vi "PH_PPPA_PowerUnit.ProcEvents.vi"(0 "i ref in":refnum<vi>, 5 "error in (no error)":errorcluster) -> (14 "i ref out":refnum<vi>, 19 "error out":errorcluster)   [LabVIEW 2014, in "PH_PPPA_PowerUnit.lvlib"]
doc: "This method is used to define the events the object will listen to. Add your own events here."
uses:
  PH_PPPA_PowerUnit.lvlib
  CS_Core/BaseProcess/BaseProcess.event definition.ctl
  CS_Core/CAEObj/CAEObj.event definition.ctl
  CS_Core/BaseProcess/BaseProcess.descriptor string definition.ctl
  PH_Basics/PH_PP_Common/PH_PP_Common.Trigger Tags.ctl
  PH_Devices/PH_Beckhoff_PP_PU/PH_Beckhoff_PP_PU.RR Tags.ctl
  PH_Basics/PH_Common/DIM/PH_DIM.Event Declarer.ctl
  PH_Devices/PH_Beckhoff_PP_Control/PH_Beckhoff_PP_Control.PP Mercury Tags.ctl
  PH_Basics/PH_PP_Common/PH_PP_Common.PSU Tags.ctl
  PH_Basics/PH_PP_Common/PH_PP_Common.PUs.ctl
  PH_Devices/PH_Beckhoff_PP_PU/PH_Beckhoff_PP_PU.Igni Tags.ctl
  CS_Core/BaseProcess/BaseProcess.lvlib
  CS_Core/CAEObj/CAEObj.lvlib
  PH_Basics/PH_Common/PH_Common.lvlib
  PH_Basics/PH_PP_Common/PH_PP_Common.lvlib
  PH_Devices/PH_Beckhoff_PP_PU/PH_Beckhoff_PP_PU.lvlib
  PH_Devices/PH_Beckhoff_PP_Control/PH_Beckhoff_PP_Control.lvlib
  PH_Basics/PH_PowerUnit_BaseClass/PH_PowerUnit_BaseClass.lvlib
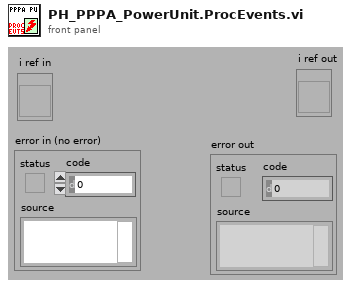
[diagram p1: front panel]
types:
  T1 = typedef "PH_Beckhoff_PP_PU.lvlib/PH_Beckhoff_PP_PU.RR Tags.ctl" = enum16{"open", "closed", "close", "Status"}
  T2 = typedef "BaseProcess.lvlib/BaseProcess.event definition.ctl" = cluster{"CAEEvtDef":T3, "Data Descriptor":T4}
  T3 = typedef "CAEObj.lvlib/CAEObj.event definition.ctl" = cluster{"URL":string, "enable":bool, "ignoreResID":bool}
  T4 = typedef "BaseProcess.lvlib/BaseProcess.descriptor string definition.ctl" = string
  T5 = typedef "PH_Common.lvlib/PH_DIM.Event Declarer.ctl" = cluster{"Service Name":string, "Selector":string}
  T6 = typedef "PH_Beckhoff_PP_Control.lvlib/PH_Beckhoff_PP_Control.PP Mercury Tags.ctl" = enum16{"Device-on", "Alarm", "on-since", "Concentration", "Status"}
  T7 = typedef "PH_PP_Common.lvlib/PH_PP_Common.PSU Tags.ctl" = enum16{"voltage-indicator", "peak-detect", "current", "voltage", "inihibit-indicator", "end-of-charge", "HV-on-indicator", "overtemperature", "interlock-indicator", "load-fault", "sum-fault", "HV-off-indicator", "DC-ok", "inhibit", "HV-on", "interlock", "reset", "Status", "Limits"}
  T8 = typedef "PH_PP_Common.lvlib/PH_PP_Common.PUs.ctl" = enum16{"no Info", "PA-19mm-1", "PA-19mm-2", "PA-45mm-PILC", "PA-45mm-MAIN", "MA-PU-1", "MA-PU-2", "MA-PU-3", "MA-PU-4", "MA-PU-5", "MA-PU-6", "MA-FR", "MA-PILC", "PA-45mm-DP"}
  T9 = typedef "PH_Beckhoff_PP_PU.lvlib/PH_Beckhoff_PP_PU.Igni Tags.ctl" = enum16{"heating-on", "water-on", "Device-on", "Status"}
  T10 = typedef "PH_PP_Common.lvlib/PH_PP_Common.Trigger Tags.ctl" = enum16{"triggered", "fired", "Status", "Last Shot"}
  T11 = typedef "PH_PowerUnit_BaseClass.lvlib/PH_PowerUnit_BaseClass.i attribute.ctl" = cluster{"Constructor finished":bool, "PU":cluster{"In use":bool, "Service ID in use":i32, "GUI Ref":refnum<vi>}, "Enabling":cluster{"State":T12, "GUI Ref":refnum<vi>}, "Timing":cluster{"Last Shot":dbl, "Time between Shots [Sec]":dbl, "Waiting Time over?":bool, "Service ID Waiting Time":i32, "GUI Ref":refnum<vi>, "Instance":cluster{"Status":T13, "linked?":bool, "GUI Ref":refnum<vi>}}, "Sequencer":cluster{"SM State":string, "GUI Ref":refnum<vi>, "linked":bool}, "Subscribed Trendmssgs":cluster{"Tagname":string, "Status":T13, "linked?":bool, "Shot Condition":T13, "GUI Ref":refnum<vi>}[], "PP PU":T8, "Default Voltage (V)":dbl, "GUI Refs":T14, "PSDB data":cluster{"Shot Voltage [V]":dbl, "State TO SM":T15, "Write 2 early":bool}, "State TO SM":T15}
  T12 = typedef "PH_SystemInformation.lvlib/PH_SystemInformationEnabling State.ctl" = i32
  T13 = typedef "PH_StatusHandler.lvlib/PH_StatusHandler.Status.ctl" = i16
  T14 = typedef "PH_PowerUnit_BaseClass.lvlib/PH_PowerUnit_BaseClass.GUI Refs.ctl" = cluster{"Delete Inst":refnum<vi>, "State TO SM":refnum<vi>, "State SM":refnum<vi>, "Fire":refnum<vi>}
  T15 = typedef "PH_PowerUnit_BaseClass.lvlib/PH_PowerUnit_BaseClass.SM States.ctl" = enum16{".", "Stand by", "Switch PU on", "Configure", "Set Default Voltage", "Set STANDBY", "Set READY", "Wait for Shot Cmd", "Open Dump Rods", "Open Ross Relais", "Close Ross Relais", "Switch PSU on", "Switch PSU off", "Charge", "Switch GD Channel on", "Close Dump Rods", "Rods-TO", "RR-TO", "PSU-TO", "Trigger-TO"}
  T16 = typedef "PH_PPPA_PowerUnit.lvlib/PH_PPPA_PowerUnit.i attribute.ctl" = cluster{"GUI Refs":cluster{"Ignitron":refnum<vi>, "Rossrelais":refnum<vi>, "Set Voltage":refnum<vi>, "PSU":refnum<vi>, "EOC":refnum<vi>, "Trigger":refnum<vi>}, "Ignitron":T17, "PSU":T18, "Dump Ross Relais":T19, "Trigger":cluster{"State Device":T13, "linked?":bool}, "Timing Settings":cluster{"Prdc Fast?":bool, "Default Value Periodic Interval":i32, "Mercury on since":dbl, "Warm up Time Mercury [s]":dbl}, "Set Voltage [V]":dbl, "19er Ignitionbox":string}
  T17 = typedef "PH_PP_Common.lvlib/PH_PP_Common.Ignitron Attributes.ctl" = cluster{"State Device":T13, "linked?":bool}
  T18 = typedef "PH_PP_Common.lvlib/PH_PP_Common.PSU Attributes.ctl" = cluster{"lower limit [V]":dbl, "upper limit [V]":dbl, "Voltage set":bool, "State Device":T13, "linked?":bool}
  T19 = typedef "PH_PP_Common.lvlib/PH_PP_Common.Ross Relais Attributes.ctl" = cluster{"State Device":T13, "linked?":bool}
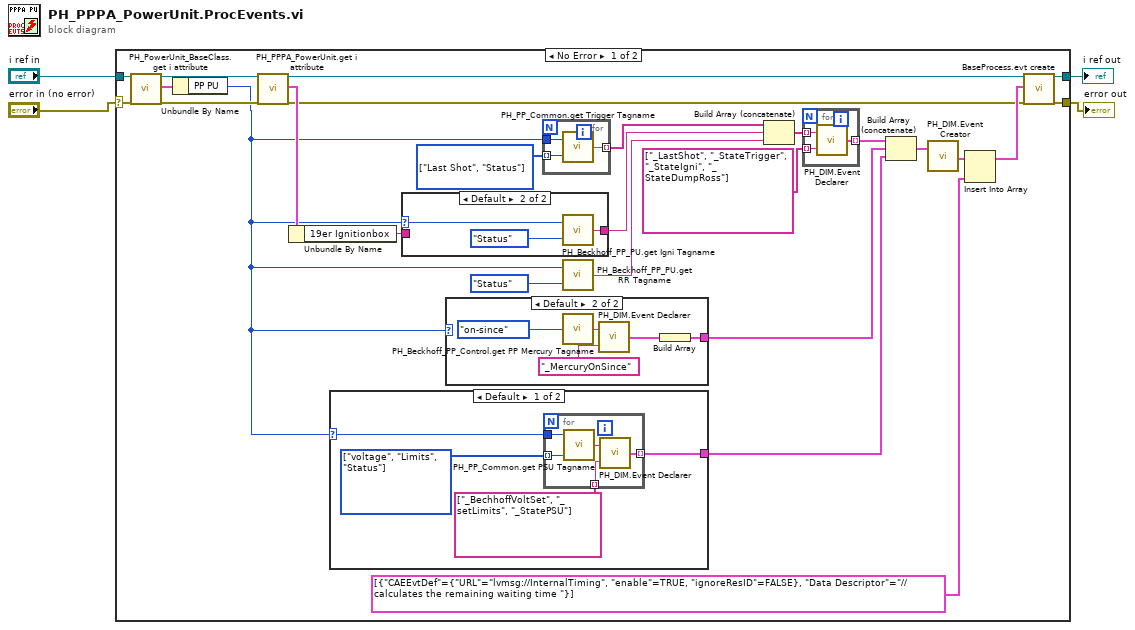
[diagram p0: block diagram]
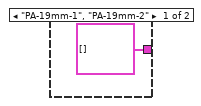
[diagram p2: hidden frame]
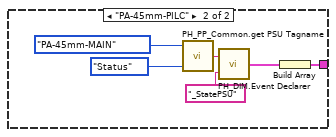
[diagram p3: hidden frame]
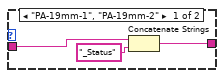
[diagram p4: hidden frame]
diagram:
  n1 = case shown="No Error" "error in (no error)" {
    selector: "error in (no error)" -> [w11 w64]
    tunnel: "i ref in" -> [w12 w65]
    tunnel: [w30 w65] -> w3
    tunnel: [w29 w64] -> w2
    frame No Error {
      w23 = T10[] [enum."Last Shot", enum."Status"] items=["triggered", "fired", "Status", "Last Shot"]
      n2 = call "PH_PowerUnit_BaseClass.get i attribute.vi"("i ref in"=w12, "error in (no error)"=w11) -> ("i ref out"=w7:refnum<vi>, "i attribute"=w6:T11, "error out"=w10:errorcluster)  [unwired: 15 in]
      n3 = Unbundle By Name(w6) -> ("PP PU"=w5:T8)
      n4 = call "PH_PPPA_PowerUnit.get i attribute.vi"("i ref in"=w7, "error in (no error)"=w10) -> ("i ref out"=w9:refnum<vi>, "i attribute"=w28:T16, "error out"=w8:errorcluster)  [unwired: 15 in]
      n5 = Unbundle By Name(w28) -> ("19er Ignitionbox"=w18:string)
      n6 = case shown="Default" w5 {
        selector: w5 -> [w38 _]
        tunnel: [w39 w46] -> w15
        frame Default {
          w40 = T7[] [enum."voltage", enum."Limits", enum."Status"] items=["voltage-indicator", "peak-detect", "current", "voltage", "inihibit-indicator", "end-of-charge", "HV-on-indicator", "overtemperature", "interlock-indicator", "load-fault", "sum-fault", "HV-off-indicator", "DC-ok", "inhibit", "HV-on", "interlock", "reset", "Status", "Limits"]
          n7 = for {
            tunnel: w38 -> [w45]
            tunnel: w40 -> [w44] mode=indexing
            tunnel: [w42] -> w39 mode=indexing
            tunnel: string[] ["_BechhoffVoltSet", "_setLimits", "_StatePSU"] -> [w41] mode=indexing
            n8 = call "PH_PP_Common.get PSU Tagname.vi"("PSU Tag"=w44, "PU"=w45) -> ("PSU Tagname"=w43:string)  [unwired: 1 in]
            n9 = call "PH_DIM.Event Declarer.vi"("Selector"=w41, "Service Name"=w43) -> ("declared DIM Event"=w42:T5)
          }
        }
        frame "PA-45mm-PILC" {
          n10 = call "PH_PP_Common.get PSU Tagname.vi"("PSU Tag"=PH_PP_Common.PSU_Tags."Status", "PU"=PH_PP_Common.PUs."PA-45mm-MAIN") -> ("PSU Tagname"=w48:string)  [unwired: 1 in]
          n11 = call "PH_DIM.Event Declarer.vi"("Selector"="_StatePSU", "Service Name"=w48) -> ("declared DIM Event"=w47:T5)
          n12 = Build Array(w47) -> (w46:T5[])
        }
      }
      n13 = case shown="Default" w5 {
        selector: w5 -> [_ w56]
        tunnel: w18 -> [w53 _]
        tunnel: [w52 w55] -> w21
        frame "PA-19mm-1", "PA-19mm-2" {
          n14 = Concatenate Strings(w53, "_Status" ("string")) -> (w52:string)
        }
        frame Default {
          n15 = call "PH_Beckhoff_PP_PU.get Igni Tagname.vi"("Igni Tag"=PH_Beckhoff_PP_PU.Igni_Tags."Status", "PU"=w56) -> ("Igni Tagname"=w55:string)
        }
      }
      n16 = case shown="Default" w5 {
        tunnel: [T5[] [] w35] -> w14
        frame "PA-19mm-1", "PA-19mm-2" {
        }
        frame Default {
          n17 = call "PH_Beckhoff_PP_Control.get PP Mercury Tagname.vi"("PP Mercury Tag"=PH_Beckhoff_PP_Control.PP_Mercury_Tags."on-since") -> ("PP Mercury Tagname"=w32:string)
          n18 = call "PH_DIM.Event Declarer.vi"("Selector"="_MercuryOnSince", "Service Name"=w32) -> ("declared DIM Event"=w36:T5)
          n19 = Build Array(w36) -> (w35:T5[])
        }
      }
      n20 = for {
        tunnel: w5 -> [w60]
        tunnel: w23 -> [w59] mode=indexing
        tunnel: [w58] -> w22 mode=indexing
        n21 = call "PH_PP_Common.get Trigger Tagname.vi"("Trigger Tag"=w59, "PU"=w60) -> ("Trigger Tagname"=w58:string)
      }
      n22 = call "PH_Beckhoff_PP_PU.get RR Tagname.vi"("Ross Relais Tag"=PH_Beckhoff_PP_PU.RR_Tags."Status", "PU"=w5) -> ("RR Tagname"=w19:string)
      n23 = Build Array (concatenate)(w22, w21, w19) -> (w24:string[])
      n24 = for {
        tunnel: w24 -> [w62] mode=indexing
        tunnel: string[] ["_LastShot", "_StateTrigger", "_StateIgni", "_StateDumpRoss"] -> [w61] mode=indexing
        tunnel: [w63] -> w17 mode=indexing
        n25 = call "PH_DIM.Event Declarer.vi"("Selector"=w61, "Service Name"=w62) -> ("declared DIM Event"=w63:T5)
      }
      n26 = Build Array (concatenate)(w17, w14, w15) -> (w16:T5[])
      n27 = call "PH_DIM.Event Creator.vi"("Trendmessage Services"=w16) -> ("DIM Service Events"=w27:T2[])  [unwired: 18 in]
      n28 = Insert Into Array(array=w27, new element=T2[] [{"CAEEvtDef"={"URL"="lvmsg://InternalTiming", "enable"=TRUE, "ignoreResID"=FALSE}, "Data Descriptor"="//calculates the remaining waiting time "}] ("new events")) -> (w25:T2[])  [unwired: 1 in]
      n29 = call "BaseProcess.evt create.vi"("i ref in"=w9, "newEvents"=w25, "error in (no error)"=w8) -> ("i ref out"=w30:refnum<vi>, "error out"=w29:errorcluster)  [unwired: 13 in, 2 out]
    }
    frame Error {
    }
  }
  "i ref out" <- w3
  "error out" <- w2
